vi "PH_Timing.PC PU in Use.vi"(0 "i ref in":refnum<vi>, 1 "Service Name":string="N/A", 2 "PU in Use?":bool, 3 "no link?":bool, 5 "error in":errorcluster) -> (14 "i ref out":refnum<vi>, 17 "PU":T1, 19 "error out":errorcluster)   [LabVIEW 2014, in "PH_Timing.lvlib"]
doc: "This VI writes the incoming information to own attributes and sets GUI elements."
uses:
  PH_Timing.lvlib
  PH_PP_Common/PH_PP_Common.PUs.ctl
  PH_PowerUnit_BaseClass/PH_PowerUnit_BaseClass.PP PU Tags.ctl
  PH_PowerUnit_BaseClass/PH_PowerUnit_BaseClass.lvlib
  PH_PP_Common/PH_PP_Common.lvlib
  PH_Common/PH_Common.lvlib
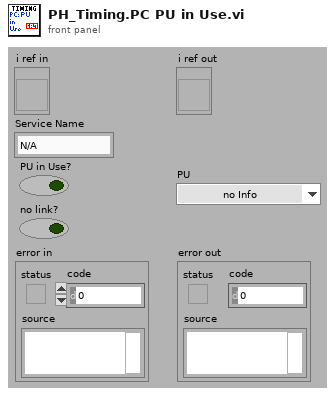
[diagram p1: front panel]
types:
  T1 = typedef "PH_PP_Common.lvlib/PH_PP_Common.PUs.ctl" = enum16{"no Info", "PA-19mm-1", "PA-19mm-2", "PA-45mm-PILC", "PA-45mm-MAIN", "MA-PU-1", "MA-PU-2", "MA-PU-3", "MA-PU-4", "MA-PU-5", "MA-PU-6", "MA-FR", "MA-PILC", "PA-45mm-DP"}
  T2 = typedef "PH_Timing.lvlib/PH_Timing.i attribute.ctl" = cluster{"Sequencer":cluster{"linked?":bool, "Proc State":string, "Ref State":refnum<vi>}, "Gate Generator":cluster{"GD":cluster{"Device Status":T3, "linked?":bool}, "Settings":T4, "GUI Ref":refnum<vi>}, "Interlock Bypass":cluster{"Instancename":string, "Switch linked?":bool, "Device Status":T3, "Ref Status":refnum<vi>}, "Roughtuner":cluster{"Settings":T5, "GUI Ref":refnum<vi>, "GD":cluster{"Device Status":T3, "linked?":bool}}, "0,5Hz Gater":cluster{"Settings":T6, "GUI Ref":refnum<vi>, "GD":cluster{"Device Status":T3, "linked?":bool}}, "Slow Trigger":cluster{"Settings":T7, "GUI Ref":refnum<vi>, "Service ID Delay":i32, "Service ID Ext Trig":i32, "Wanted Settings":T7}, "Timing Mode":cluster{"Mode":T8, "GUI Ref":refnum<vi>, "Service ID T2":i32, "Service ID Mode":i32, "Wanted Mode":T8}, "ns Generator":cluster{"Settings":T9, "ns Generator Settings":refnum<vi>, "GD":cluster{"Device Status":T3, "linked?":bool}}, "Phase FEs":cluster{"Settings":T12, "GUI Ref":refnum<vi>, "Service ID Phase":i32, "Wanted Settings":T12}, "GD GUI Refs":refnum<vi>[], "Heads":T13[], "GUI Ref Delete":refnum<vi>}
  T3 = typedef "PH_StatusHandler.lvlib/PH_StatusHandler.Status.ctl" = i16
  T4 = typedef "PH_Timing.lvlib/PH_Timing.GateGen.ctl" = cluster{"Instance":string, "Channel Gate":i32, "Channel T2":i32, "Width Gate":dbl, "Width T2":dbl, "Delay Gate":dbl, "Delay T2":dbl, "Gate activ":bool, "T2 activ":bool, "System Mode":enum16{"Normal", "Single", "Burst", "Duty Cycle"}}
  T5 = typedef "PH_Timing.lvlib/PH_Timing.Roughtuner.ctl" = cluster{"Instance":string, "Phase PHELIX / UNILAC":cluster{"Channel":u16, "relative to":u16, "Delay [ms]":dbl}, "Pulse Length":cluster{"Channel":u16, "relative to":u16, "Delay [ms]":dbl}, "Trigger":cluster{"externally?":bool, "Rate [Hz]":dbl}}
  T6 = typedef "PH_Timing.lvlib/PH_Timing.0.5HzGater.ctl" = cluster{"Instance":string, "Channel ns FE Delay":i32, "Channel 0.5Hz":i32, "Width ns FE Delay":dbl, "Width 0.5Hz":dbl, "Delay ns FE Delay":dbl, "Delay 0.5Hz":dbl, "ns FE Delay active":bool, "0.5Hz activ":bool, "ns FE Delay inverted":bool, "0.5Hz inverted":bool}
  T7 = typedef "PH_Timing.lvlib/PH_Timing.Slow Trigger Settings.ctl" = cluster{"Delay":dbl, "externally triggered?":bool}
  T8 = typedef "PH_Timing.lvlib/PH_Timing.Timing Mode.ctl" = cluster{"T2":i16, "Modeselector":enum32{"10 Hz", "0.5 Hz", "Shot"}}
  T9 = typedef "PH_Timing.lvlib/PH_Timing.ns Generator.ctl" = cluster{"Instance":string, "Phase fs / ns FE":cluster{"Channel":T10, "Settings":T11}}
  T10 = typedef "Stanford Research DG645 - Driver.lvlib/Channel.ctl" = i32
  T11 = typedef "PH_SRDG645.lvlib/PH_SRDG645.Channel Settings.ctl" = cluster{"Delay [s]":dbl, "relative to":i32}
  T12 = typedef "PH_Timing.lvlib/PH_Timing.Phase FEs.ctl" = cluster{"Phase":dbl}
  T13 = typedef "PH_Timing.lvlib/PH_Timing.PU Data.ctl" = cluster{"linked?":bool, "Data":T14, "GD":cluster{"Device Status":T3, "linked?":bool}, "GUI Ref":refnum<vi>, "PU":T1}
  T14 = typedef "PH_Timing.lvlib/PH_Timing.PU Info.ctl" = cluster{"Act CH?":bool, "GD":string, "CH":i32, "Delay":dbl, "active":bool, "in Use?":bool}
  T15 = typedef "PH_PowerUnit_BaseClass.lvlib/PH_PowerUnit_BaseClass.PP PU Tags.ctl" = enum16{"Waiting-Time", "PU-in-Use"}
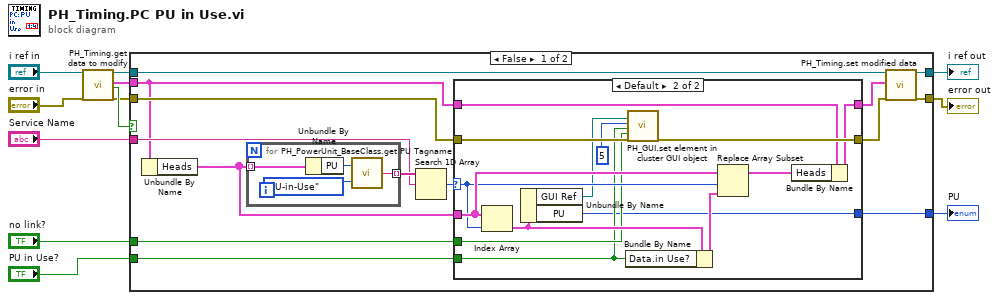
[diagram p0: block diagram]
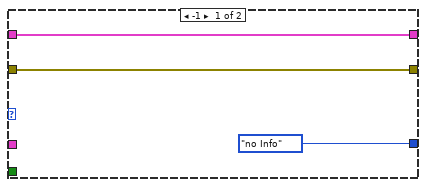
[diagram p2: hidden frame]
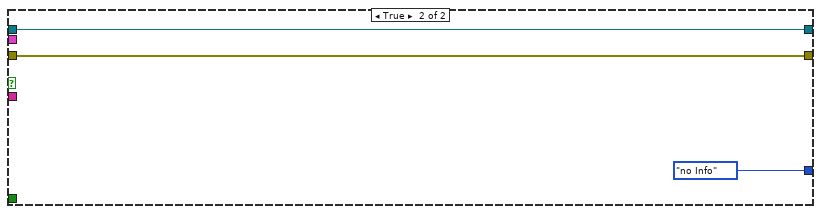
[diagram p3: hidden frame]
diagram:
  n1 = call "PH_Timing.get data to modify.vi"("i ref in"="i ref in", "error in (no error)"="error in") -> ("i ref out"=w9:refnum<vi>, "i attribute"=w11:T2, "timed out"=w12:bool, "error out"=w10:errorcluster)  [unwired: 14 in]
  n2 = case shown="False" w12 {
    tunnel: w9 -> [w17 w50]
    tunnel: [w26 w50] -> w3
    tunnel: w10 -> [w24 w49]
    tunnel: [w25 w49] -> w2
    tunnel: w11 -> [w15 _]
    tunnel: "no link?" -> [w14 _]
    tunnel: "Service Name" -> [w18 _]
    tunnel: "PU in Use?" -> [w21 _]
    tunnel: [w16 PH_PP_Common.PUs."no Info" ("PU")] -> w1
    frame False {
      n3 = Unbundle By Name(w15) -> ("Heads"=w13:T13[])
      n4 = for {
        tunnel: w13 -> [w30] mode=indexing
        tunnel: [w27] -> w19 mode=indexing
        n5 = Unbundle By Name(w30) -> ("PU"=w29:T1)
        n6 = call "PH_PowerUnit_BaseClass.get PU Tagname.vi"("PU Tag"=PH_PowerUnit_BaseClass.PP_PU_Tags."PU-in-Use", "PU"=w29) -> ("PU Tagname"=w27:string)
      }
      n7 = Search 1D Array(1D array=w19, element=w18) -> (index of element=w20:i32)  [unwired: 1 in]
      n8 = case shown="Default" w20 {
        selector: w20 -> [_ w40]
        tunnel: w24 -> [w33 w47]
        tunnel: [w33 w46] -> w23
        tunnel: w14 -> [_ w39]
        tunnel: w21 -> [_ w36]
        tunnel: w15 -> [w32 w45]
        tunnel: [w32 w44] -> w22
        tunnel: w13 -> [_ w42]
        tunnel: [PH_PP_Common.PUs."no Info" ("PU") w35] -> w16
        frame -1 {
        }
        frame Default {
          n9 = Index Array(array=w42, index=w40) -> (element=w43:T13)
          n10 = Unbundle By Name(w43) -> ("GUI Ref"=w37:refnum<vi>, "PU"=w35:T1)
          n11 = Bundle By Name(cluster=w43, "Data.in Use?"=w36) -> (w41:T13)
          n12 = call "PH_GUI.set element in cluster GUI object.vi"("Cluster Ref"=w37, "Cluster index"=5, "Value"=w36, "Blinking? (false)"=w39, "error in (no error)"=w47) -> ("error out"=w46:errorcluster)  [unwired: 14 in]
          n13 = Replace Array Subset(array=w42, new element=w41, index=w40) -> (w34:T13[])
          n14 = Bundle By Name(cluster=w45, "Heads"=w34) -> (w44:T2)
        }
      }
      n15 = call "PH_Timing.set modified data.vi"("i ref in"=w17, "i attribute"=w22, "error in (no error)"=w23) -> ("i ref out"=w26:refnum<vi>, "error out"=w25:errorcluster)  [unwired: 15 in]
    }
    frame True {
    }
  }
  "error out" <- w2
  "i ref out" <- w3
  "PU" <- w1
